vi "Recieve TCP_IP Message.vi"(8 "error in (no error)":errorcluster, 10 "timeout ms (25000)":i32=25000, 11 "WebSocket in":refnum<class "WebSocket.lvclass">) -> (0 "error out":errorcluster, 2 "Message":string, 3 "WebSocket out":refnum<class "WebSocket.lvclass">)   [LabVIEW 2024, in "Ramses Framework.lvlib"]
doc: "Reads an incoming message using **#** header format, where # is a U64 representing message size."
uses:
  Ramses Framework.lvlib
  <vilib>/MediaMongrels Ltd/WebSockets/WebSockets/WebSocket/WebSocket.lvclass
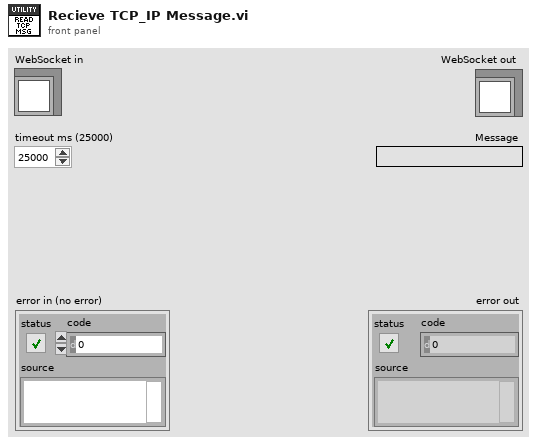
[diagram p1: front panel]
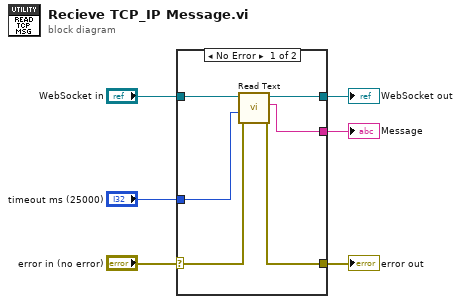
[diagram p0: block diagram]
diagram:
  n1 = case shown="No Error" "error in (no error)" {
    selector: "error in (no error)" -> [w8 w13]
    tunnel: [w12 w13] -> w6
    tunnel: [w11 w14] -> w5
    tunnel: "WebSocket in" -> [w10 w14]
    tunnel: "timeout ms (25000)" -> [w9 _]
    tunnel: [w7 _] -> w4
    frame No Error {
      n2 = call-dynamic "Read Text.vi"("error in (no error)"=w8, "timeout ms (5000)"=w9, "WebSocket in"=w10) -> ("error out"=w12:errorcluster, "Data"=w7:string, "WebSocket out"=w11:refnum<class "WebSocket.lvclass">)  [unwired: 6 in]
    }
    frame Error {
    }
  }
  "error out" <- w6
  "WebSocket out" <- w5
  "Message" <- w4
